vi "to string 1.0.vi"(8 "error in (no error)":errorcluster, 10 "data in":string, 11 "Sequencer Module configuration in":refnum<class "Sequencer Module configuration.lvclass">) -> (0 "error out":errorcluster, 2 "data out":string, 3 "Sequencer Module configuration out":refnum<class "Sequencer Module configuration.lvclass">)   [LabVIEW 2015, in "Sequencer Module configuration.lvclass"]
uses:
  Sequencer Module configuration.lvclass
  Sequencer Module configuration.lvclass/Sequencer Module configuration.ctl
  classes/Sequence/Config/Sequence Config.lvclass
  <vilib>/NI/Configuration Framework/serializable configuration/NISE_CEF_serializable configuration.lvclass
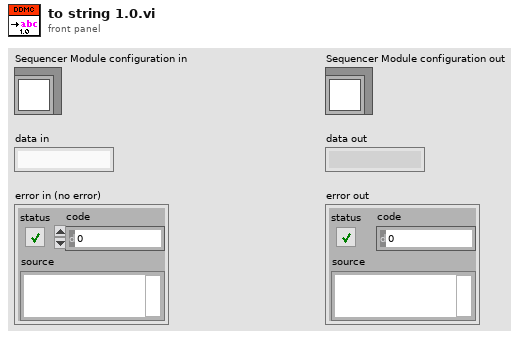
[diagram p1: front panel]
types:
  T1 = typedef "Sequencer Module configuration.lvclass/Line.ctl" = cluster{"Sequence":refnum<class "Sequence Config.lvclass">}
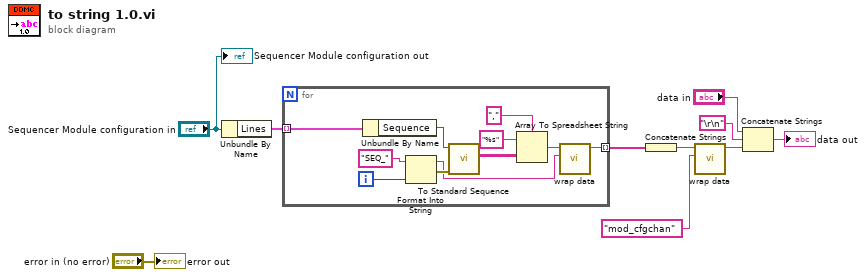
[diagram p0: block diagram]
diagram:
  n1 = Unbundle By Name("Sequencer Module configuration in") -> ("Lines"=w2:T1[])
  n2 = for {
    tunnel: w2 -> [w21] mode=indexing
    tunnel: [w13] -> w1 mode=indexing
    i -> [w18]
    n3 = Unbundle By Name(w21) -> ("Sequence"=w20:refnum<class "Sequence Config.lvclass">)
    n4 = Format Into String(initial string="SEQ_", w18) -> (resulting string=w16:string, error out=w19:errorcluster)  [unwired: 2 in]
    n5 = call-dynamic "To Standard Sequence.vi"("error in (no error)"=w19, "Sequence Config in"=w20) -> ("Standard Sequence"=w12:string[][])  [unwired: 7 in, 2 out]
    n6 = Array To Spreadsheet String(delimiter (Tab)=",", array=w12, 3:"%s" ("format string")) -> (spreadsheet string=w14:string)
    n7 = call <vilib>:"wrap data.vi"("identifier"=w16, "data to wrap"=w14) -> ("wrapped data"=w13:string)  [unwired: 9 in]
  }
  n8 = Concatenate Strings(w1) -> (w4:string)
  n9 = call <vilib>:"wrap data.vi"("identifier"="mod_cfgchan", "data to wrap"=w4) -> ("wrapped data"=w8:string)  [unwired: 9 in]
  n10 = Concatenate Strings("data in", "\r\n", w8) -> (→"data out":string)
  "error out" <- "error in (no error)"
  "Sequencer Module configuration out" <- "Sequencer Module configuration in"
